vi "publishFPGAData.vi"(8 "error in (no error)":errorcluster, 11 "Telemetry in":refnum<class "Telemetry.lvclass">) -> (0 "error out":errorcluster, 3 "Telemetry out":refnum<class "Telemetry.lvclass">)   [LabVIEW 2016, in "Telemetry.lvclass"]
uses:
  Telemetry.lvclass
  Telemetry.lvclass/Telemetry.ctl
  UserEvents/UserEvents.lvclass
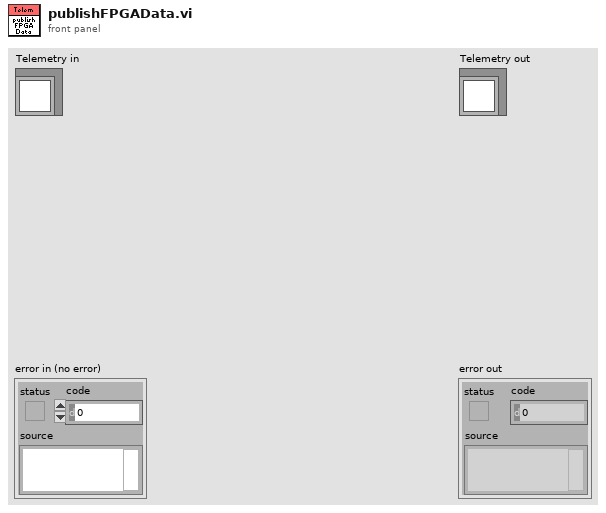
[diagram p1: front panel]
types:
  T1 = typedef "M1M3Communicator.lvlib/TelemetryFPGAData.ctl" = cluster{"Timestamp":T2, "ModbusSubnetATxInternalFIFOOverflow":bool, "ModbusSubnetAInvalidInstruction":bool, "ModbusSubnetAWaitForRxFrameTimeout":bool, "ModbusSubnetAStartBitError":bool, "ModbusSubnetAStopBitError":bool, "ModbusSubnetARxDataFIFOOverflow":bool, "ModbusSubnetATxByteCount":i32, "ModbusSubnetATxFrameCount":i32, "ModbusSubnetARxByteCount":i32, "ModbusSubnetARxFrameCount":i32, "ModbusSubnetBTxInternalFIFOOverflow":bool, "ModbusSubnetBInvalidInstruction":bool, "ModbusSubnetBWaitForRxFrameTimeout":bool, "ModbusSubnetBStartBitError":bool, "ModbusSubnetBStopBitError":bool, "ModbusSubnetBRxDataFIFOOverflow":bool, "ModbusSubnetBTxByteCount":i32, "ModbusSubnetBTxFrameCount":i32, "ModbusSubnetBRxByteCount":i32, "ModbusSubnetBRxFrameCount":i32, "ModbusSubnetCTxInternalFIFOOverflow":bool, "ModbusSubnetCInvalidInstruction":bool, "ModbusSubnetCWaitForRxFrameTimeout":bool, "ModbusSubnetCStartBitError":bool, "ModbusSubnetCStopBitError":bool, "ModbusSubnetCRxDataFIFOOverflow":bool, "ModbusSubnetCTxByteCount":i32, "ModbusSubnetCTxFrameCount":i32, "ModbusSubnetCRxByteCount":i32, "ModbusSubnetCRxFrameCount":i32, "ModbusSubnetDTxInternalFIFOOverflow":bool, "ModbusSubnetDInvalidInstruction":bool, "ModbusSubnetDWaitForRxFrameTimeout":bool, "ModbusSubnetDStartBitError":bool, "ModbusSubnetDStopBitError":bool, "ModbusSubnetDRxDataFIFOOverflow":bool, "ModbusSubnetDTxByteCount":i32, "ModbusSubnetDTxFrameCount":i32, "ModbusSubnetDRxByteCount":i32, "ModbusSubnetDRxFrameCount":i32, "ModbusSubnetETxInternalFIFOOverflow":bool, "ModbusSubnetEInvalidInstruction":bool, "ModbusSubnetEWaitForRxFrameTimeout":bool, "ModbusSubnetEStartBitError":bool, "ModbusSubnetEStopBitError":bool, "ModbusSubnetERxDataFIFOOverflow":bool, "ModbusSubnetETxByteCount":i32, "ModbusSubnetETxFrameCount":i32, "ModbusSubnetERxByteCount":i32, "ModbusSubnetERxFrameCount":i32, "FPGATimestamp":dbl}
  T2 = typedef "M1M3SupportTypes.lvlib/Timestamp.ctl" = dbl
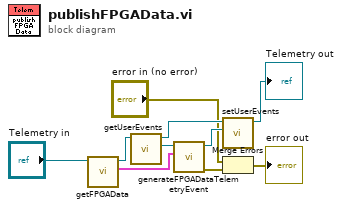
[diagram p0: block diagram]
diagram:
  n1 = call "getFPGAData.vi"("Telemetry in"="Telemetry in") -> ("TelemetryFPGAData"=w8:T1, "Telemetry out"=w9:refnum<class "Telemetry.lvclass">)  [unwired: 9 in]
  n2 = call "getUserEvents.vi"("Telemetry in"=w9) -> ("UserEvents"=w7:refnum<class "UserEvents.lvclass">, "Telemetry out"=w5:refnum<class "Telemetry.lvclass">)  [unwired: 9 in]
  n3 = call "generateFPGADataTelemetryEvent.vi"("TelemetryFPGAData"=w8, "UserEvents in"=w7) -> ("error out"=w3:errorcluster, "UserEvents out"=w6:refnum<class "UserEvents.lvclass">)  [unwired: 8 in]
  n4 = call "setUserEvents.vi"("UserEvents"=w6, "Telemetry in"=w5) -> ("Telemetry out"=→"Telemetry out":refnum<class "Telemetry.lvclass">)  [unwired: 9 in]
  n5 = Merge Errors("error in (no error)", w3) -> (→"error out":errorcluster)
